vi "FMS Data Array.vi"() -> (0 "FMS Data Array":string[](array[string]))   [LabVIEW 2017]
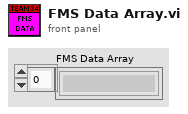
[diagram p1: front panel]
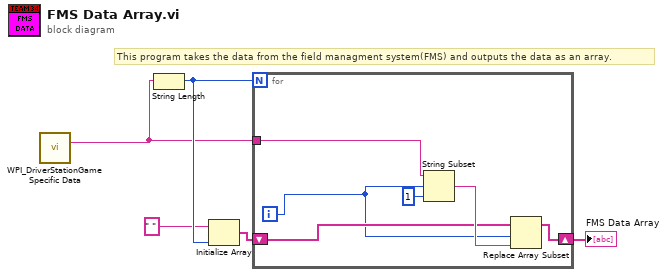
[diagram p0: block diagram]
diagram:
  # "This program takes the data from the field managment system(FMS) and outputs the data as an array."
  n1 = call <vilib>:"WPI_DriverStationGame Specific Data.vi"() -> ("Game Specific Data"=w2:string)  [unwired: 11 in]
  n2 = String Length(string=w2) -> (length=w5:i32)
  n3 = Initialize Array(" ", w5) -> (w3:string[])
  n4 = for {
    N: w5 -> [_]
    shift-right: [w8] -> w1
    shift-left: w3 -> [w9]
    tunnel: w2 -> [w6]
    i -> [w7]
    n5 = String Subset(string=w6, offset (0)=w7, length (rest)=1 ("length (rest)")) -> (substring=w10:string)
    n6 = Replace Array Subset(array=w9, new element=w10, index=w7) -> (w8:string[])
  }
  "FMS Data Array" <- w1
